vi "MGI Handle New Row(s).vi"(8 "error in (no error)":errorcluster, 10 "NewRows[]":i32[](array[numeric]), 11 "Error Reporter Dialog in":refnum<class "MGI Error Reporter Dialog.lvclass">) -> (0 "error out":errorcluster, 3 "Error Reporter Dialog out":refnum<class "MGI Error Reporter Dialog.lvclass">)   [LabVIEW 2020, in "MGI Error Reporter Dialog.lvclass"]
doc: "Handles UI Updates necessary when new error row(s) are added to the error reporter dialog's Listbox. A child class may override this VI, which calls ShowUI. <B>NewRows[]</B> contains the indices of the inserted rows.\n\n\nAuthored by Shawn Walpole\nsupport@mooregoodideas.com\nwww.mooregoodideas.com\n\nCopyright (c) 2010, Moore Good Ideas, Inc.\n\nAll rights reserved.\n\nRedistribution and use in source and binary forms, with or without modification, are permitted provided that the following conditions are met:\n\n * Redistributions of source code must retain the above copyright notice, this list of conditions and the following disclaimer.\n * Redistributions in binary form must reproduce the above copyright notice, this list of conditions and the following disclaimer in the documentation and/or other materials provided with the distribution.\n * Neither the name of Moore Good Ideas, Inc. nor the names of its contributors may be used to endorse or promote products derived from this software without specific prior written permission.\n\nTHIS SOFTWARE IS PROVIDED BY THE COPYRIGHT HOLDERS AND CONTRIBUTORS \"AS IS\" AND ANY EXPRESS OR IMPLIED WARRANTIES, INCLUDING, BUT NOT LIMITED TO, THE IMPLIED WARRANTIES OF MERCHANTABILITY AND FITNESS FOR A PARTICULAR PURPOSE ARE DISCLAIMED. IN NO EVENT SHALL THE COPYRIGHT OWNER OR CONTRIBUTORS BE LIABLE FOR ANY DIRECT, INDIRECT, INCIDENTAL, SPECIAL, EXEMPLARY, OR CONSEQUENTIAL DAMAGES (INCLUDING, BUT NOT LIMITED TO, PROCUREMENT OF SUBSTITUTE GOODS OR SERVICES; LOSS OF USE, DATA, OR PROFITS; OR BUSINESS INTERRUPTION) HOWEVER CAUSED AND ON ANY THEORY OF LIABILITY, WHETHER IN CONTRACT, STRICT LIABILITY, OR TORT (INCLUDING NEGLIGENCE OR OTHERWISE) ARISING IN ANY WAY OUT OF THE USE OF THIS SOFTWARE, EVEN IF ADVISED OF THE POSSIBILITY OF SUCH DAMAGE."
uses:
  <userlib>/_MGI/Error Reporter/MGI Error Reporter Dialog/MGI Error Reporter Dialog.lvclass
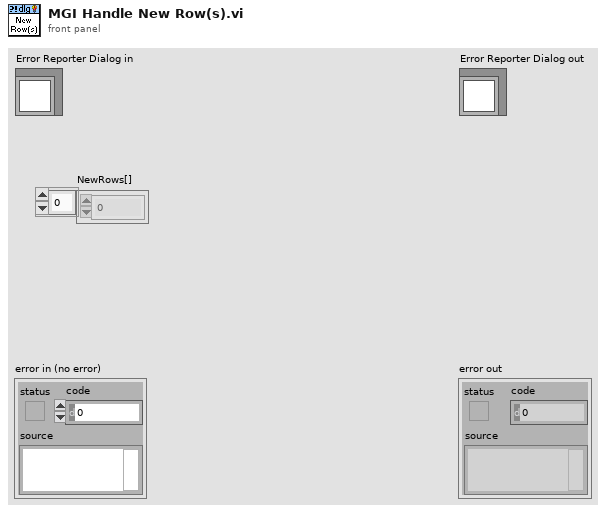
[diagram p1: front panel]
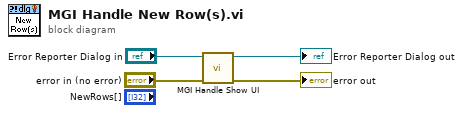
[diagram p0: block diagram]
diagram:
  n1 = call-dynamic "MGI Handle Show UI.vi"("error in (no error)"="error in (no error)", "MGI Error Reporter Dialog In"="Error Reporter Dialog in") -> ("error out"=→"error out":errorcluster, "MGI Error Reporter Dialog Out"=→"Error Reporter Dialog out":refnum<class "MGI Error Reporter Dialog.lvclass">)  [unwired: 8 out]
